vi "Deadband.vi"(1 "Axes":dbl[](array[numeric])) -> (0 "Deadbanded Axes":dbl[](array[numeric]))   [LabVIEW 2018]
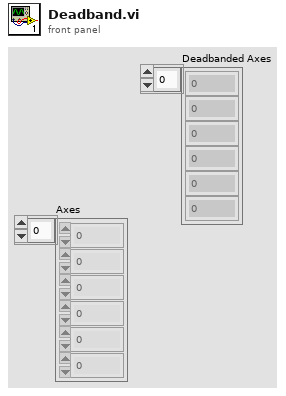
[diagram p1: front panel]
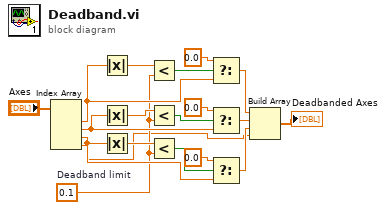
[diagram p0: block diagram]
diagram:
  w6 = 0.1  # Deadband limit
  n1 = Index Array(array="Axes") -> (element #1=w9:dbl, element #2=w8:dbl, element #3=w7:dbl, element #4=w1:dbl)  [unwired: 4 in]
  n2 = Absolute Value(x=w9) -> (abs(x)=w16:dbl)
  n3 = Absolute Value(x=w8) -> (abs(x)=w13:dbl)
  n4 = Absolute Value(x=w7) -> (abs(x)=w10:dbl)
  n5 = Less?(x=w16, y=w6) -> (x < y?=w17:bool)
  n6 = Less?(x=w13, y=w6) -> (x < y?=w14:bool)
  n7 = Less?(x=w10, y=w6) -> (x < y?=w11:bool)
  n8 = Select(t=0.0, s=w17, f=w9) -> (s? t:f=w5:dbl)
  n9 = Select(t=0.0, s=w14, f=w8) -> (s? t:f=w4:dbl)
  n10 = Select(t=0.0, s=w11, f=w7) -> (s? t:f=w3:dbl)
  n11 = Build Array(w5, w4, w3, w1) -> (→"Deadbanded Axes":dbl[])
